vi "save_read_device_config.vi"(2 "w-r":enum16{"save", "read"}(ring), 3 "intput table":string[][](array[string])=[["dede", ""], ["", "ddddd"]]) -> (0 "error out":errorcluster, 1 "output table":string[][](array[string]))   [LabVIEW 2026]
uses:
  <vilib>/Utility/NIReport.llb/Report Type.ctl
  <vilib>/Utility/file.llb/Write Delimited Spreadsheet (string).vi
  <vilib>/Utility/NIReport.llb/Append Text Table to Report (wrap).vi
  <vilib>/Utility/file.llb/Read Delimited Spreadsheet (string).vi
  <vilib>/addons/_office/excel.llb/Excel Get Data ([str]).vi
  <vilib>/Utility/NIReport.llb/NI_report.lvclass
  <vilib>/Utility/NIReport.llb/NI_ReportGenerationCore.lvlib
  <vilib>/Utility/NIReport.llb/Excel/NI_Excel.lvclass
  <vilib>/addons/_office/NI_ReportGenerationToolkit.lvlib
panel:
  in  "csv-excel":enum16{"csv", "excel"}(ring)
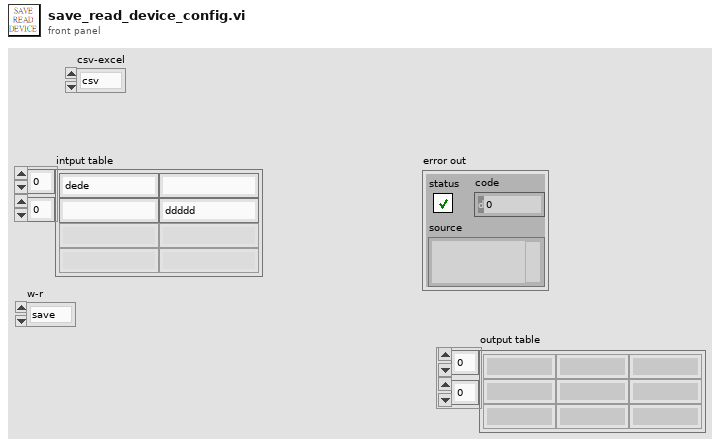
[diagram p1: front panel]
types:
  T1 = typedef "NI_ReportGenerationCore.lvlib/Report Type.ctl" = enum16{"HTML", "Word", "Excel"}
  T2 = enum16{"maximized", "minimized", "normal", "no change"}
  T3 = enum16{"Standard Report", "HTML", "Word", "Excel"}
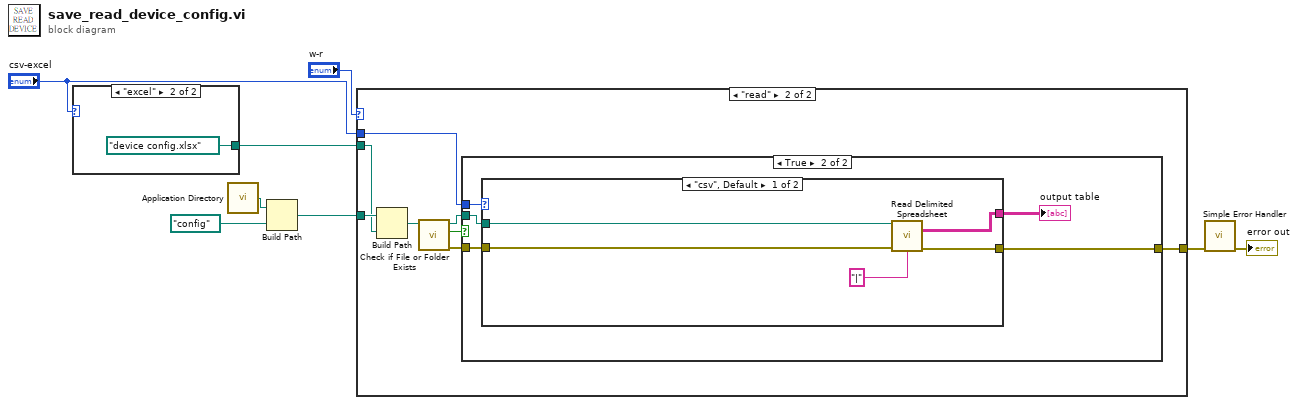
[diagram p0: block diagram]
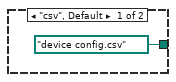
[diagram p2: hidden frame]
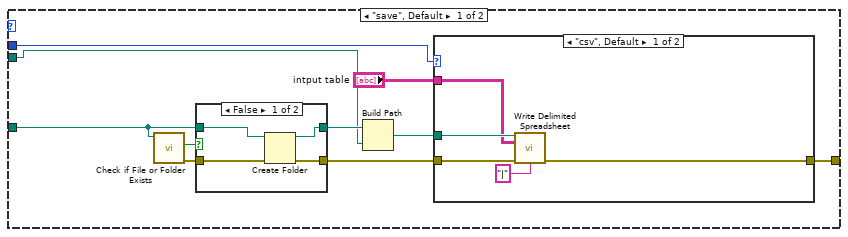
[diagram p3: hidden frame]
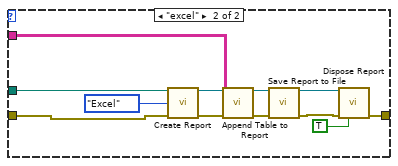
[diagram p4: hidden frame]
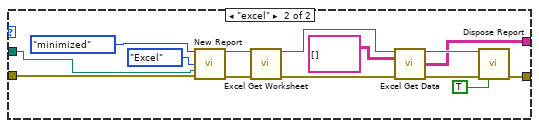
[diagram p7: hidden frame]
diagram:
  n1 = case shown="\"excel\"" "csv-excel" {
    tunnel: [path "device config.csv" ("name or relative path") path "device config.xlsx" ("name or relative path")] -> w2
    frame "csv", Default {
    }
    frame "excel" {
    }
  }
  n2 = call <vilib>:"Application Directory.vi"() -> ("Application Directory"=w8:path)
  n3 = Build Path(base path=w8, name or relative path=path "config") -> (appended path=w6:path)
  n4 = case shown="\"read\"" "w-r" {
    tunnel: w2 -> [w16 w46]
    tunnel: w6 -> [w15 w47]
    tunnel: [w14 w45] -> w5
    tunnel: "csv-excel" -> [w11 w44]
    frame "save", Default {
      n5 = call <vilib>:"Check if File or Folder Exists.vi"("path"=w15) -> ("error out"=w13:errorcluster, "file or folder exists?"=w17:bool)  [unwired: 8 in, 1 out]
      n6 = case shown="False" w17 {
        tunnel: w15 -> [w41 w43]
        tunnel: [w40 w43] -> w18
        tunnel: w13 -> [w39 w42]
        tunnel: [w38 w42] -> w12
        frame False {
          n7 = Create Folder(path (use dialog)=w41, error in=w39) -> (created path=w40:path, error out=w38:errorcluster)  [unwired: 1 in, 1 out]
        }
        frame True {
        }
      }
      n8 = Build Path(base path=w18, name or relative path=w16) -> (appended path=w19:path)
      n9 = case shown="\"csv\", Default" w11 {
        tunnel: "intput table" -> [w24 w37]
        tunnel: w19 -> [w25 w30]
        tunnel: [w22 w27] -> w14
        tunnel: w12 -> [w23 w26]
        frame "csv", Default {
          n10 = call-poly <vilib>:"Write Delimited Spreadsheet.vi"("file path (dialog if empty)"=w25, "2D data"=w24, "error in (no error)"=w23, "delimiter (\\t)"="|" ("delimiter (\\t)")) -> ("error out"=w22:errorcluster)  [unwired: 10 in, 1 out]
        }
        frame "excel" {
          n11 = call <vilib>:"Create Report.vi"("report type"=Report_Type."Excel" ("Report Type"), "error in (no error)"=w26) -> ("report out"=w32:refnum<class "NI_report.lvclass">, "error out"=w31:errorcluster)  [unwired: 12 in]
          n12 = call-poly <vilib>:"Append Table to Report.vi"("report in"=w32, "text data"=w37, "error in (no error)"=w31) -> ("report out"=w33:refnum<class "NI_report.lvclass">, "error out"=w34:errorcluster)  [unwired: 9 in, 2 out]
          n13 = call-dynamic "Save Report to File.vi"("report in"=w33, "report file path"=w30, "error in (no error)"=w34) -> ("report out"=w36:refnum<class "NI_report.lvclass">, "error out"=w35:errorcluster)  [unwired: 11 in]
          n14 = call-dynamic "Dispose Report.vi"("report in"=w36, "error in (no error)"=w35, "close report? (T)"=TRUE ("Close Report? (T)")) -> ("error out"=w27:errorcluster)  [unwired: 12 in]
        }
      }
    }
    frame "read" {
      n15 = Build Path(base path=w47, name or relative path=w46) -> (appended path=w48:path)
      n16 = call <vilib>:"Check if File or Folder Exists.vi"("path"=w48) -> ("error out"=w51:errorcluster, "file or folder exists?"=w49:bool, "dup path"=w50:path)  [unwired: 8 in]
      n17 = case shown="True" w49 {
        tunnel: [w52 w57] -> w45
        tunnel: w50 -> [_ w56]
        tunnel: w51 -> [w52 w55]
        tunnel: w44 -> [_ w54]
        frame False {
        }
        frame True {
          n18 = case shown="\"csv\", Default" w54 {
            tunnel: [w60 w72] -> w57
            tunnel: w56 -> [w58 w68]
            tunnel: w55 -> [w59 w66]
            tunnel: [w61 w63] -> w53
            frame "csv", Default {
              n19 = call-poly <vilib>:"Read Delimited Spreadsheet.vi"("file path (dialog if empty)"=w58, "error in (no error)"=w59, "delimiter (\\t)"="|" ("delimiter (\\t)")) -> ("all rows"=w61:string[][], "error out"=w60:errorcluster)  [unwired: 7 in, 4 out]
            }
            frame "excel" {
              n20 = call <vilib>:"New Report.vi"("window state (normal)"=T2."minimized", "report type"=T3."Excel", "template (empty)"=w68, "error in (no error)"=w66) -> ("report out"=w75:refnum<class "NI_report.lvclass">, "error out"=w65:errorcluster)  [unwired: 10 in]
              n21 = call <vilib>:"Excel Get Worksheet.vi"("report in"=w75, "error in (no error)"=w65) -> ("report out"=w74:refnum<class "NI_report.lvclass">, "error out"=w64:errorcluster)  [unwired: 12 in]
              n22 = call-poly <vilib>:"Excel Get Data.vi"("report in"=w74, "data type"=string[][] [], "error in (no error)"=w64) -> ("report out"=w70:refnum<class "NI_report.lvclass">, "data"=w63:string[][], "error out"=w69:errorcluster)  [unwired: 10 in]
              n23 = call-dynamic "Dispose Report.vi"("report in"=w70, "error in (no error)"=w69, "close report? (T)"=TRUE ("Close Report? (T)")) -> ("error out"=w72:errorcluster)  [unwired: 12 in]
            }
          }
          "output table" <- w53
        }
      }
    }
  }
  n24 = call <vilib>:"Simple Error Handler.vi"("error in (no error)"=w5) -> ("error out"=→"error out":errorcluster)  [unwired: 4 in, 4 out]
